vi "Connect.vi"(6 "error in":errorcluster, 7 "Address":string, 9 "RawSocket Handler in":refnum<class "RawSocket TCP Handler.lvclass">) -> (0 "error out":errorcluster, 3 "RawSocket Handler out":refnum<class "RawSocket TCP Handler.lvclass">)   [LabVIEW 2020, in "wamplv.lvlib" / "RawSocket TCP Handler.lvclass"]
uses:
  RawSocket TCP Handler.lvclass
  <vilib>/LabVIEW Open Source Project/OpenURI/uri/URI.lvclass
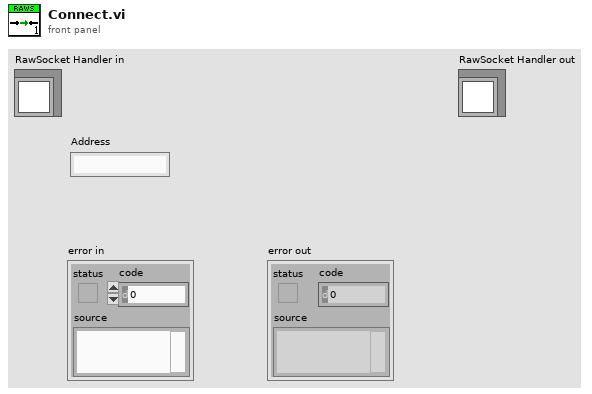
[diagram p1: front panel]
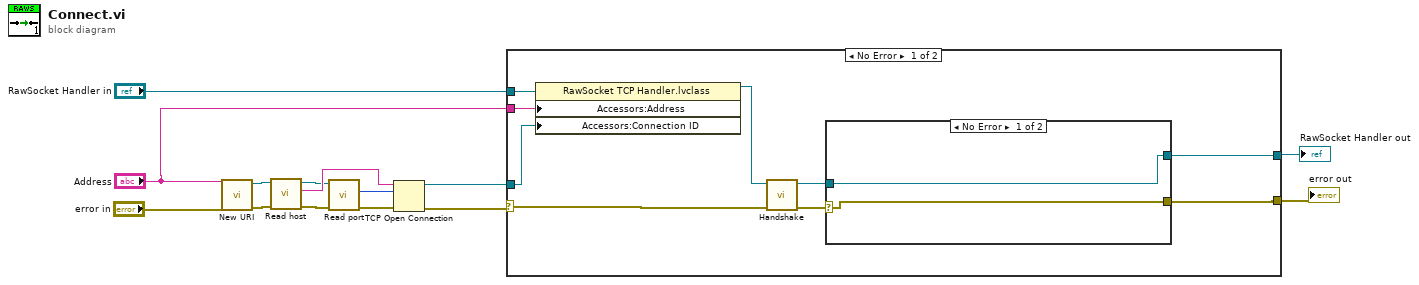
[diagram p0: block diagram]
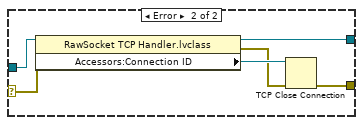
[diagram p2: hidden frame]
diagram:
  n1 = call <vilib>:"New URI.vi"("error in (no error)"="error in", "URI"="Address") -> ("error out"=w11:errorcluster, "URI"=w12:refnum<class "URI.lvclass">)  [unwired: 8 in]
  n2 = call <vilib>:"Read host.vi"("error in (no error)"=w11, "URI in"=w12) -> ("error out"=w9:errorcluster, "host"=w10:string, "URI out"=w8:refnum<class "URI.lvclass">)  [unwired: 7 in]
  n3 = call <vilib>:"Read port.vi"("error in (no error)"=w9, "URI in"=w8) -> ("error out"=w5:errorcluster, "port"=w7:u16)  [unwired: 7 in, 1 out]
  n4 = TCP Open Connection(address=w10, remote port or service name=w7, error in (no error)=w5) -> (connection ID=w4:refnum<k5>, error out=w1:errorcluster)  [unwired: 2 in]
  n5 = case shown="No Error" w1 {
    selector: w1 -> [w15 w33]
    tunnel: "RawSocket Handler in" -> [w23 w32]
    tunnel: "Address" -> [w22 _]
    tunnel: w4 -> [w19 _]
    tunnel: [w18 w33] -> w3
    tunnel: [w16 w32] -> w2
    frame No Error {
      n6 = property class="RawSocket TCP Handler.lvclass"(reference=w23, "Accessors:Address"=w22, "Accessors:Connection ID"=w19) -> (reference out=w21:refnum<class "RawSocket TCP Handler.lvclass">)  [unwired: 1 in, 1 out]
      n7 = call "Handshake.vi"("error in"=w15, "RawSocket Handler in"=w21) -> ("error out"=w20:errorcluster, "RawSocket Handler out"=w17:refnum<class "RawSocket TCP Handler.lvclass">)  [unwired: 8 in]
      n8 = case shown="No Error" w20 {
        selector: w20 -> [w25 w28]
        tunnel: [w25 w31] -> w18
        tunnel: w17 -> [w24 w30]
        tunnel: [w24 w26] -> w16
        frame No Error {
        }
        frame Error {
          n9 = property class="RawSocket TCP Handler.lvclass"(reference=w30, error in=w28) -> (reference out=w26:refnum<class "RawSocket TCP Handler.lvclass">, error out=w27:errorcluster, "Accessors:Connection ID"=w29:refnum<k5>)
          n10 = TCP Close Connection(connection ID=w29, error in (no error)=w27) -> (error out=w31:errorcluster)  [unwired: 1 in, 1 out]
        }
      }
    }
    frame Error {
    }
  }
  "RawSocket Handler out" <- w2
  "error out" <- w3
